vi "ezAFM Practice 1.2.vi"() -> ()   [LabVIEW 2015]
uses:
  D:/LabVIEW for ezAFM/LV-PGC 2019-05a/Special Equipment/ezAFM/NMI Integration Code/ezCommander.dll
  LabVIEW for ezAFM/LV-PGC 2019-05a/Special Equipment/ezAFM/NMI Integration Code/ezCommander.dll
  LabVIEW for ezAFM/LV-PGC 2019-05a/Universal vi's/Global Variables/Globals-EasyAFM.vi
panel:
  in  "File Path":path
  out "Scanning":bool
  in  "ABORT SCAN":bool
  in  "BEGIN SCAN":bool
  out "Retracting":bool
  out "Approaching":bool
  in  "APPROACH":bool
  out "XYZ Motor Position":dbl[](array[numeric])
  in  "RETRACT":bool
  out "XY Vector":dbl[](array[numeric])
  in  "Target Device":string(combo)
  in  "Current Device":string(combo)
  in  "MOVE":bool
  in  "THETA":bool
  in  "Angle":dbl
  in  "RESET":bool
  out "ezAFM Connected":bool
  in  "QUIT":bool
  out "XY Position":dbl[](array[numeric])
  out "Status":dbl
  in  "Step Size":dbl
  in  "Motor Speed":dbl
  in  "LEFT":bool
  in  "RIGHT":bool
  in  "DOWN":bool
  in  "UP":bool
  # "Use Arrow Keys to Navigate\nXY Motor"
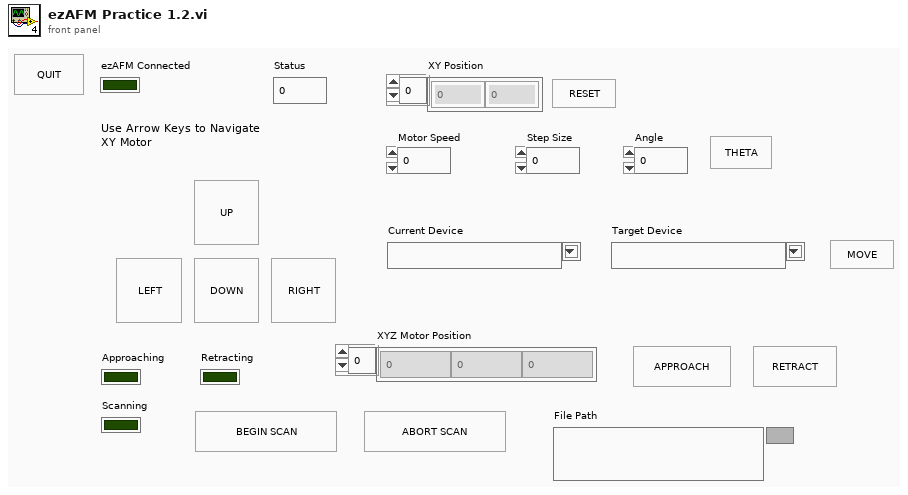
[diagram p1: front panel]
types:
  T1 = enum16{"Read XYZ Motor Position", "Read XYZ Piezo Position", "Read Setpoint", "Begin AutoLand", "Begin AutoLand, Wait till done", "XYZ Motions", "Init Scan (from global settings)", "Start Scan", "Stop Scan"}
  T2 = cluster{"Approach":bool, "Retract":bool, "Up":bool, "Up-Right":bool, "Right":bool, "Up Left":bool}
  T3 = typedef "eventvkey.ctl" = enum16{"ASCII", "Enter", "Return", "Shift", "Ctrl", "Alt", "Cmd", "Opt", "Caps", "NumLock", "Clear", "Break", "Up", "Down", "Left", "Right", "Insert", "Delete", "Home", "End", "PageUp", "PageDown", "Escape", "Help", "Pause", "ScrollLock", "F1", "F2", "F3", "F4", "F5", "F6", "F7", "F8", "F9", "F10", "F11", "F12", "F13", "F14", "F15", "F16", "F17", "F18", "F19", "F20", "F21", "F22", "F23", "F24", "Play", "VolumeUp", "VolumeDown", "Mute", "Two Byte Char"}
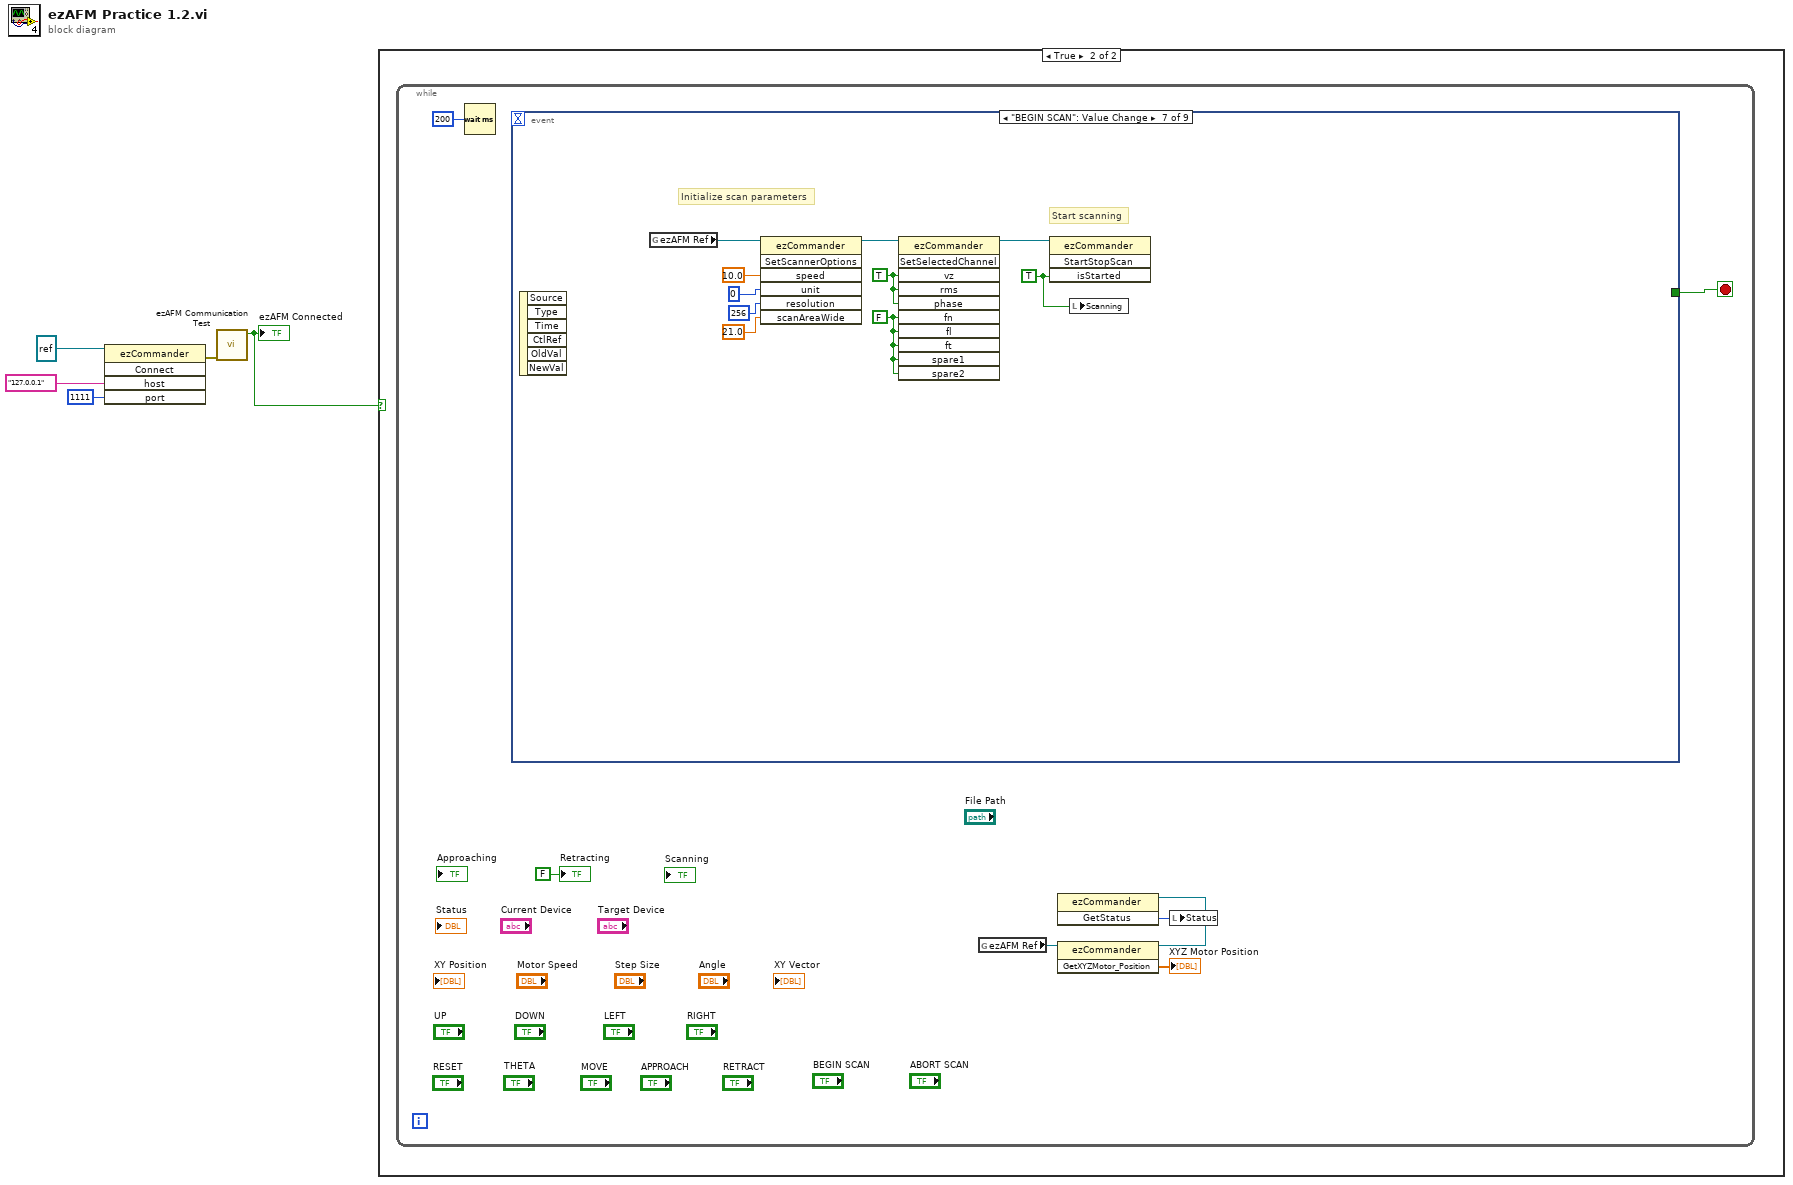
[diagram p0: block diagram]
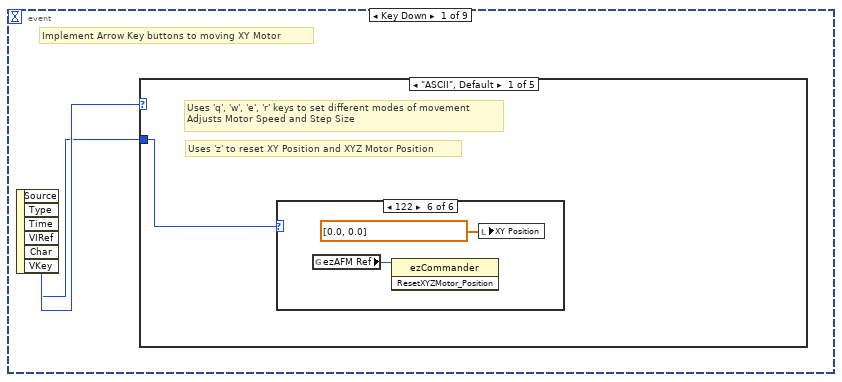
[diagram p3: hidden frame]
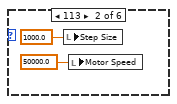
[diagram p5: hidden frame]
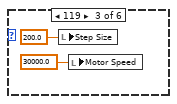
[diagram p6: hidden frame]
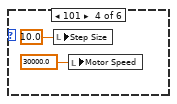
[diagram p7: hidden frame]
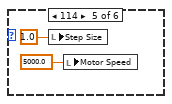
[diagram p8: hidden frame]
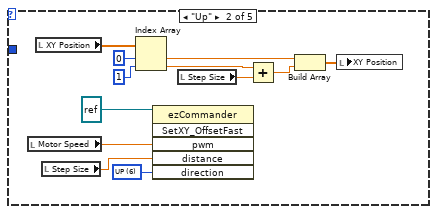
[diagram p9: hidden frame]
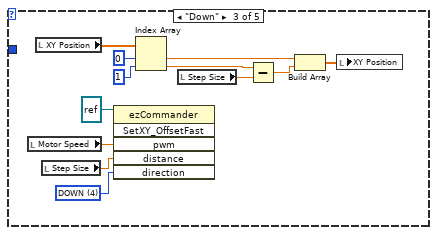
[diagram p10: hidden frame]
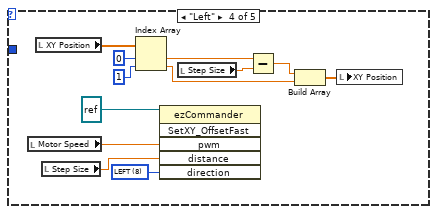
[diagram p11: hidden frame]
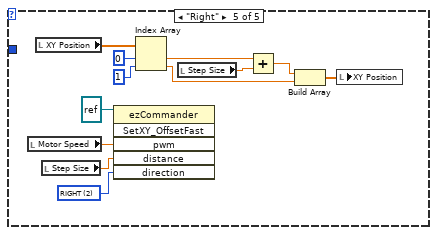
[diagram p12: hidden frame]
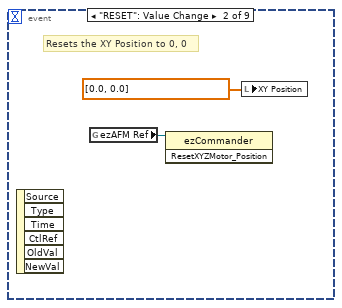
[diagram p13: hidden frame]
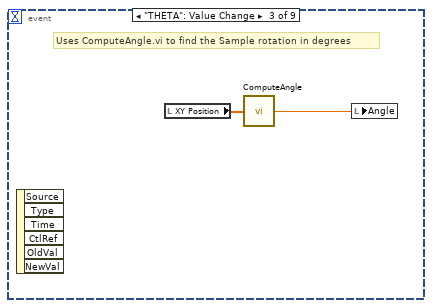
[diagram p14: hidden frame]
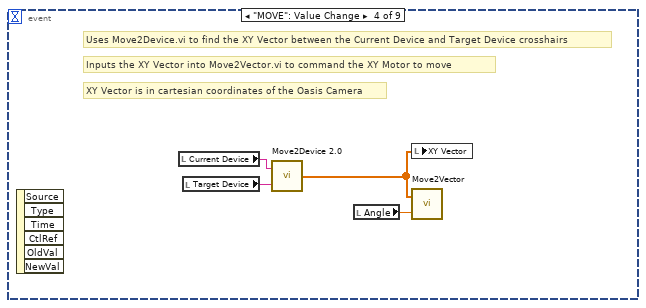
[diagram p15: hidden frame]
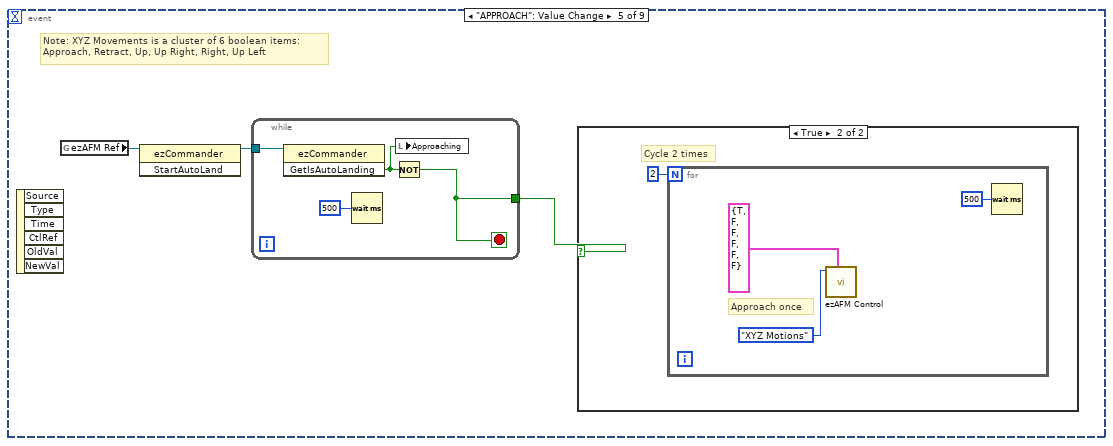
[diagram p16: hidden frame]
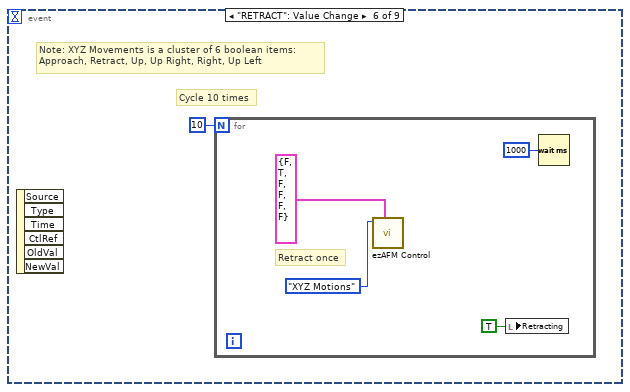
[diagram p18: hidden frame]
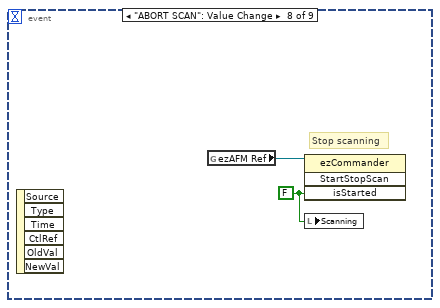
[diagram p19: hidden frame]
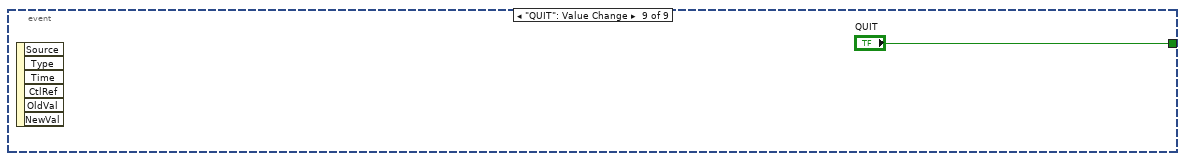
[diagram p20: hidden frame]
diagram:
  n1 = invoke class="ezCommander" method="Connect"(reference=refnum<k24> refnum ("ezAFM Ref"), "host"="127.0.0.1", "port"=1111) -> (error out=w4:errorcluster)  [unwired: 2 in, 4 out]
  n2 = call "ezAFM Communication Test.vi"("error in"=w4) -> ("ezAFM COM status"=w1:bool)  [unwired: 3 in, 3 out]
  "ezAFM Connected" <- w1
  n3 = case shown="True" w1 {
    frame False {
    }
    frame True {
      n4 = while {
        stop <- w11 stop-if-true
        n5 = Wait (ms)(milliseconds to wait=u32 200) -> ()  [unwired: 1 out]
        n6 = event shown="[6] \"BEGIN SCAN\": Value Change" {
          selector: _ -> [_ _ _ _ _ _ _ _ _]
          dyn-events: _ -> [_ _ _ _ _ _ _ _ _]
          timeout: _ -> [_ _ _ _ _ _ _ _ _]
          tunnel: [_ _ _ _ _ _ _ _ "QUIT"] -> w11
          event Key Down {
            # "Implement Arrow Key buttons to moving XY Motor"
            n7 = event-data() -> ("Char"=w12:i16, "VKey"=w13:T3)  [unwired: 1 in, 4 out]
            n8 = case shown="\"ASCII\", Default" w13 {
              tunnel: w12 -> [w14 _ _ _ _]
              frame "ASCII", Default {
                # "Uses 'z' to reset XY Position and XYZ Motor Position"
                # "Uses 'q', 'w', 'e', 'r' keys to set different modes of movement\nAdjusts Motor Speed and Step Size"
                n9 = case shown="122" w14 {
                  frame 0, Default {
                  }
                  frame 113 {
                    n10 = local write "Step Size"(1000.0 ("Step Size")) -> ()
                    n11 = local write "Motor Speed"(50000.0 ("Motor Speed")) -> ()
                  }
                  frame 119 {
                    n12 = local write "Step Size"(200.0 ("Step Size")) -> ()
                    n13 = local write "Motor Speed"(30000.0 ("Motor Speed")) -> ()
                  }
                  frame 101 {
                    n14 = local write "Step Size"(10.0 ("Step Size")) -> ()
                    n15 = local write "Motor Speed"(30000.0 ("Motor Speed")) -> ()
                  }
                  frame 114 {
                    n16 = local write "Step Size"(1.0 ("Step Size")) -> ()
                    n17 = local write "Motor Speed"(5000.0 ("Motor Speed")) -> ()
                  }
                  frame 122 {
                    n18 = global read "Globals-EasyAFM.vi" "ezAFM Ref"() -> (w23:refnum<k24>)
                    n19 = invoke class="ezCommander" method="ResetXYZMotor_Position"(reference=w23) -> ()  [unwired: 2 in, 3 out]
                    n20 = local write "XY Position"(dbl[] [0.0, 0.0] ("XY Position")) -> ()
                  }
                }
              }
              frame "Up" {
                w35 = u16 6 items=["UP"=6, "DOWN"=4, "LEFT"=8, "RIGHT"=2]
                n21 = local read "Motor Speed"() -> (w34:dbl)
                n22 = local read "XY Position"() -> (w32:dbl[])
                n23 = local read "Step Size"() -> (w33:dbl)
                n24 = Index Array(array=w32, index #1=0 ("index"), index #2=1 ("index")) -> (element #1=w27:dbl, element #2=w28:dbl)
                n25 = invoke class="ezCommander" method="SetXY_OffsetFast"(reference=refnum<k24> refnum ("ezAFM Ref"), "pwm"=w34, "distance"=w33, "direction"=w35) -> ()  [unwired: 2 in, 6 out]
                n26 = local read "Step Size"() -> (w29:dbl)
                n27 = Add(x=w28, y=w29) -> (x+y=w26:dbl)
                n28 = Build Array(w27, w26) -> (w25:dbl[])
                n29 = local write "XY Position"(w25) -> ()
              }
              frame "Down" {
                w45 = u16 4 items=["UP"=6, "DOWN"=4, "LEFT"=8, "RIGHT"=2]
                n30 = local read "Motor Speed"() -> (w47:dbl)
                n31 = local read "XY Position"() -> (w39:dbl[])
                n32 = local read "Step Size"() -> (w46:dbl)
                n33 = invoke class="ezCommander" method="SetXY_OffsetFast"(reference=refnum<k24> refnum ("ezAFM Ref"), "pwm"=w47, "distance"=w46, "direction"=w45) -> ()  [unwired: 2 in, 6 out]
                n34 = Index Array(array=w39, index #1=0 ("index"), index #2=1 ("index")) -> (element #1=w41:dbl, element #2=w42:dbl)
                n35 = local read "Step Size"() -> (w38:dbl)
                n36 = Subtract(x=w42, y=w38) -> (x-y=w40:dbl)
                n37 = Build Array(w41, w40) -> (w37:dbl[])
                n38 = local write "XY Position"(w37) -> ()
              }
              frame "Left" {
                w59 = u16 8 items=["UP"=6, "DOWN"=4, "LEFT"=8, "RIGHT"=2]
                n39 = local read "Motor Speed"() -> (w57:dbl)
                n40 = local read "XY Position"() -> (w53:dbl[])
                n41 = local read "Step Size"() -> (w58:dbl)
                n42 = Index Array(array=w53, index #1=0 ("index"), index #2=1 ("index")) -> (element #1=w51:dbl, element #2=w49:dbl)
                n43 = invoke class="ezCommander" method="SetXY_OffsetFast"(reference=refnum<k24> refnum ("ezAFM Ref"), "pwm"=w57, "distance"=w58, "direction"=w59) -> ()  [unwired: 2 in, 6 out]
                n44 = local read "Step Size"() -> (w54:dbl)
                n45 = Subtract(x=w51, y=w54) -> (x-y=w50:dbl)
                n46 = Build Array(w50, w49) -> (w52:dbl[])
                n47 = local write "XY Position"(w52) -> ()
              }
              frame "Right" {
                w71 = u16 2 items=["UP"=6, "DOWN"=4, "LEFT"=8, "RIGHT"=2]
                n48 = local read "Motor Speed"() -> (w70:dbl)
                n49 = local read "XY Position"() -> (w65:dbl[])
                n50 = local read "Step Size"() -> (w69:dbl)
                n51 = invoke class="ezCommander" method="SetXY_OffsetFast"(reference=refnum<k24> refnum ("ezAFM Ref"), "pwm"=w70, "distance"=w69, "direction"=w71) -> ()  [unwired: 2 in, 6 out]
                n52 = Index Array(array=w65, index #1=0 ("index"), index #2=1 ("index")) -> (element #1=w63:dbl, element #2=w61:dbl)
                n53 = local read "Step Size"() -> (w64:dbl)
                n54 = Add(x=w63, y=w64) -> (x+y=w62:dbl)
                n55 = Build Array(w62, w61) -> (w66:dbl[])
                n56 = local write "XY Position"(w66) -> ()
              }
            }
          }
          event "RESET": Value Change {
            # "Resets the XY Position to 0, 0"
            n57 = event-data() -> ()  [unwired: 1 in, 6 out]
            n58 = global read "Globals-EasyAFM.vi" "ezAFM Ref"() -> (w73:refnum<k24>)
            n59 = invoke class="ezCommander" method="ResetXYZMotor_Position"(reference=w73) -> ()  [unwired: 2 in, 3 out]
            n60 = local write "XY Position"(dbl[] [0.0, 0.0] ("XY Position")) -> ()
          }
          event "THETA": Value Change {
            # "Uses ComputeAngle.vi to find the Sample rotation in degrees"
            n61 = event-data() -> ()  [unwired: 1 in, 6 out]
            n62 = local read "XY Position"() -> (w76:dbl[])
            n63 = call "ComputeAngle.vi"("XY Vector"=w76) -> ("Angle"=w75:dbl)
            n64 = local write "Angle"(w75) -> ()
          }
          event "MOVE": Value Change {
            # "XY Vector is in cartesian coordinates of the Oasis Camera"
            # "Inputs the XY Vector into Move2Vector.vi to command the XY Motor to move"
            # "Uses Move2Device.vi to find the XY Vector between the Current Device and Target Device crosshairs"
            n65 = event-data() -> ()  [unwired: 1 in, 6 out]
            n66 = local read "Current Device"() -> (w79:string)
            n67 = local read "Target Device"() -> (w78:string)
            n68 = call "Move2Device 2.0.vi"("Target Device"=w78, "Current Device"=w79) -> ("XY Vector"=w77:dbl[])
            n69 = local read "Angle"() -> (w80:dbl)
            n70 = local write "XY Vector"(w77) -> ()
            n71 = call "Move2Vector.vi"("Angle"=w80, "XY Vector"=w77) -> ()  [unwired: 1 in]
          }
          event "APPROACH": Value Change {
            # "Note: XYZ Movements is a cluster of 6 boolean items: \nApproach, Retract, Up, Up Right, Right, Up Left"
            n72 = event-data() -> ()  [unwired: 1 in, 6 out]
            n73 = global read "Globals-EasyAFM.vi" "ezAFM Ref"() -> (w82:refnum<k24>)
            n74 = invoke class="ezCommander" method="StartAutoLand"(reference=w82) -> (reference out=w83:refnum<k24>)  [unwired: 2 in, 2 out]
            n75 = while {
              tunnel: w83 -> [w91]
              tunnel: [w88] -> w81
              stop <- w88 stop-if-true
              n76 = invoke class="ezCommander" method="GetIsAutoLanding"(reference=w91) -> ("GetIsAutoLanding"=w90:bool)  [unwired: 2 in, 2 out]
              n77 = Wait (ms)(milliseconds to wait=u32 500) -> ()  [unwired: 1 out]
              n78 = Not(x=w90) -> (.not. x?=w88:bool)
              n79 = local write "Approaching"(w90) -> ()
            }
            n80 = case shown="True" w81 {
              frame False {
              }
              frame True {
                # "Cycle 2 times"
                n81 = for {
                  N: 2 -> [_]
                  # "Approach once"
                  n82 = call "ezAFM Control.vi"("XYZ Movements"=T2 {"Approach"=TRUE, "Retract"=FALSE, "Up"=FALSE, "Up-Right"=FALSE, "Right"=FALSE, "Up Left"=FALSE}, "Mode"=T1."XYZ Motions") -> ()  [unwired: 3 in, 4 out]
                  n83 = Wait (ms)(milliseconds to wait=u32 500) -> ()  [unwired: 1 out]
                }
              }
            }
          }
          event "RETRACT": Value Change {
            # "Cycle 10 times"
            # "Note: XYZ Movements is a cluster of 6 boolean items: \nApproach, Retract, Up, Up Right, Right, Up Left"
            n84 = event-data() -> ()  [unwired: 1 in, 6 out]
            n85 = for {
              N: 10 -> [_]
              # "Retract once"
              n86 = call "ezAFM Control.vi"("XYZ Movements"=T2 {"Approach"=FALSE, "Retract"=TRUE, "Up"=FALSE, "Up-Right"=FALSE, "Right"=FALSE, "Up Left"=FALSE}, "Mode"=T1."XYZ Motions") -> ()  [unwired: 3 in, 4 out]
              n87 = local write "Retracting"(TRUE ("Retracting")) -> ()
              n88 = Wait (ms)(milliseconds to wait=u32 1000) -> ()  [unwired: 1 out]
            }
          }
          event "BEGIN SCAN": Value Change {
            w99 = FALSE
            w100 = TRUE
            w106 = TRUE ("isStarted")
            # "Start scanning"
            # "Initialize scan parameters"
            n89 = event-data() -> ()  [unwired: 1 in, 6 out]
            n90 = global read "Globals-EasyAFM.vi" "ezAFM Ref"() -> (w98:refnum<k24>)
            n91 = invoke class="ezCommander" method="SetScannerOptions"(reference=w98, "speed"=10.0, "unit"=0, "resolution"=256, "scanAreaWide"=21.0) -> (reference out=w97:refnum<k24>)  [unwired: 2 in, 6 out]
            n92 = invoke class="ezCommander" method="SetSelectedChannel"(reference=w97, "vz"=w100, "rms"=w100, "phase"=w100, "fn"=w99, "fl"=w99, "ft"=w99, "spare1"=w99, "spare2"=w99) -> (reference out=w105:refnum<k24>)  [unwired: 2 in, 10 out]
            n93 = invoke class="ezCommander" method="StartStopScan"(reference=w105, "isStarted"=w106) -> ()  [unwired: 2 in, 4 out]
            n94 = local write "Scanning"(w106) -> ()
          }
          event "ABORT SCAN": Value Change {
            w107 = FALSE ("isStarted")
            # "Stop scanning"
            n95 = event-data() -> ()  [unwired: 1 in, 6 out]
            n96 = global read "Globals-EasyAFM.vi" "ezAFM Ref"() -> (w108:refnum<k24>)
            n97 = invoke class="ezCommander" method="StartStopScan"(reference=w108, "isStarted"=w107) -> ()  [unwired: 2 in, 4 out]
            n98 = local write "Scanning"(w107) -> ()
          }
          event "QUIT": Value Change {
            n99 = event-data() -> ()  [unwired: 1 in, 6 out]
          }
        }
        n100 = global read "Globals-EasyAFM.vi" "ezAFM Ref"() -> (w6:refnum<k24>)
        n101 = invoke class="ezCommander" method="GetStatus"(reference=w6) -> ("GetStatus"=w8:i32)  [unwired: 2 in, 2 out]
        n102 = invoke class="ezCommander" method="GetXYZMotor_Position"(reference=w6) -> ("GetXYZMotor_Position"=→"XYZ Motor Position":dbl[])  [unwired: 2 in, 2 out]
        n103 = local write "Status"(w8) -> ()
        "Retracting" <- FALSE ("Retracting")
      }
    }
  }
